vi "Create Title.vi"(10 "Font":T1, 11 "Title":string) -> (2 "Title Box Size":cluster{"Width":u32, "Height":u32}, 3 "Title out":picture)   [LabVIEW 2018, in "PieChart.lvclass"]
uses:
  PieChart.lvclass
  <vilib>/picture/picture.llb/Draw True-Color Pixmap.vi
  <vilib>/Utility/miscctls.llb/LVFontTypeDef.ctl
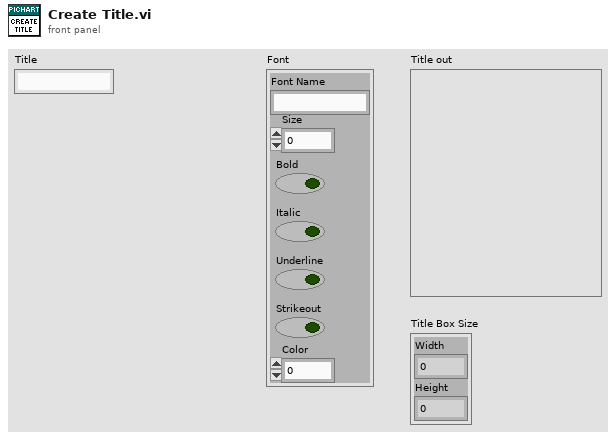
[diagram p1: front panel]
types:
  T1 = typedef "LVFontTypeDef.ctl" = cluster{"Font Name":string, "Size":u16, "Bold":bool, "Italic":bool, "Underline":bool, "Strikeout":bool, "Color":u32}
  T2 = cluster{"left":i16, "top":i16, "right":i16, "bottom":i16}
  T3 = enum16{"User-specified Font", "Application Font", "System Font", "Dialog Font"}
  T4 = cluster{"Font Name:":string, "Size":i16, "Strikeout?":bool, "Italic?":bool, "Underline?":bool, "Outline?":bool, "Shadow?":bool, "Bold?":bool}
  T5 = cluster{"left":u32, "top":u32, "right":u32, "bottom":u32}
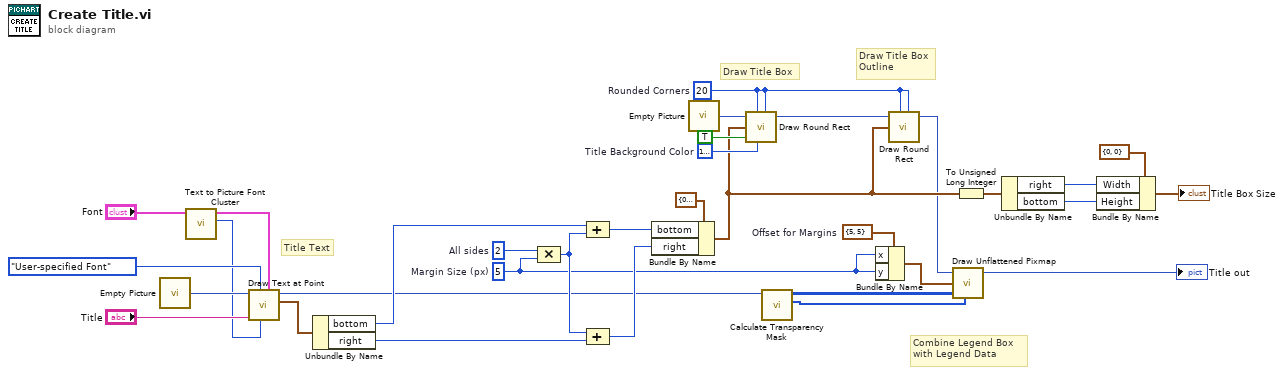
[diagram p0: block diagram]
diagram:
  w7 = i16 20  # Rounded Corners
  w23 = i16 2  # All sides
  w21 = cluster{"x":i16, "y":i16} {"x"=5, "y"=5}  # Offset for Margins
  w29 = u32 16777238  # Title Background Color
  w19 = i16 5  # Margin Size (px)
  # "Title Text"
  # "Draw Title Box"
  # "Combine Legend Box\nwith Legend Data"
  # "Draw Title Box\nOutline"
  n1 = call "Empty Picture"() -> ("empty picture"=w26:picture)
  n2 = call "Text to Picture Font Cluster.vi"("Text Font Cluster"="Font") -> ("Color"=w4:u32, "Picture Font Cluster"=w5:T4)  [unwired: 9 in]
  n3 = call <vilib>:"Draw Text at Point.vi"("[user-specified font]"=w5, "text color(black)"=w4, "desired font(Application)"=T3."User-specified Font", "text"="Title", "picture"=w26) -> ("text rect"=w11:T2, "new picture"=w3:picture)  [unwired: 5 in]
  n4 = Unbundle By Name(w11) -> ("bottom"=w9:i16, "right"=w8:i16)
  n5 = Compound Arithmetic op=MULTIPLY(w23, w19) -> (w22:i16)
  n6 = Compound Arithmetic op=ADD(w9, w22) -> (w31:i16)
  n7 = Compound Arithmetic op=ADD(w22, w8) -> (w24:i16)
  n8 = Bundle By Name(cluster=T2 {"left"=0, "top"=0, "right"=0, "bottom"=0} ("rect"), "bottom"=w31, "right"=w24) -> (w17:T2)
  n9 = call "Empty Picture"() -> ("empty picture"=w25:picture)
  n10 = call <vilib>:"Draw Round Rect.vi"("picture"=w25, "oval width"=w7, "rect"=w17, "fill?(F)"=TRUE, "color(black)"=w29, "oval height"=w7) -> ("new picture"=w28:picture)  [unwired: 3 in]
  n11 = call "Calculate Transparency Mask.vi"("Picture in"=w3) -> ("mask"=w1:u8[], "24-bit pixmap"=w2:u32[][])  [unwired: 8 in, 1 out]
  n12 = Bundle By Name(cluster=w21, "x"=w19, "y"=w19) -> (w20:cluster{"x":i16, "y":i16})
  n13 = call <vilib>:"Draw Round Rect.vi"("picture"=w28, "oval width"=w7, "rect"=w17, "oval height"=w7) -> ("new picture"=w12:picture)  [unwired: 5 in]
  n14 = call-poly <vilib>:"Draw Unflattened Pixmap.vi"("picture"=w12, "top left point(0, 0)"=w20, "data (RGB format)"=w2, "mask"=w1) -> ("new picture"=→"Title out":picture)  [unwired: 5 in]
  n15 = To Unsigned Long Integer(number=w17) -> (unsigned 32bit integer=w13:T5)
  n16 = Unbundle By Name(w13) -> ("right"=w16:u32, "bottom"=w14:u32)
  n17 = Bundle By Name(cluster=cluster{"Width":u32, "Height":u32} {"Width"=0, "Height"=0} ("Legend Box Size"), "Width"=w16, "Height"=w14) -> (→"Title Box Size":cluster{"Width":u32, "Height":u32})
